vi "Filter.vi"(7 "Bandwidth":i32=2, 8 "error in (no error)":errorcluster, 9 "Frequency":i32=2, 10 "Channel index":i32=2, 11 "array":waveform(dbl)[](array[waveform])) -> (0 "error out":errorcluster, 1 "dt":dbl, 2 "Channel name":string, 3 "Amplitude":dbl)   [LabVIEW 2019]
doc: "This example demonstrates how to acquire a continuous amount of data (Waveform) using the DAQ device's internal clock. It also shows how to synchronize two devices for different device families (E Series, S Series, M Series, X Series, DSA, and SC Express), to simultaneously acquire the data.\n\nFor instructions on how to connect your signals to the DAQ device, refer to your device documentation."
uses:
  <vilib>/Waveform/WDTOps.llb/WDT Get Final Time Value DBL.vi
  <vilib>/Analysis/NI_AALPro.lvlib
panel:
  # "Filter"
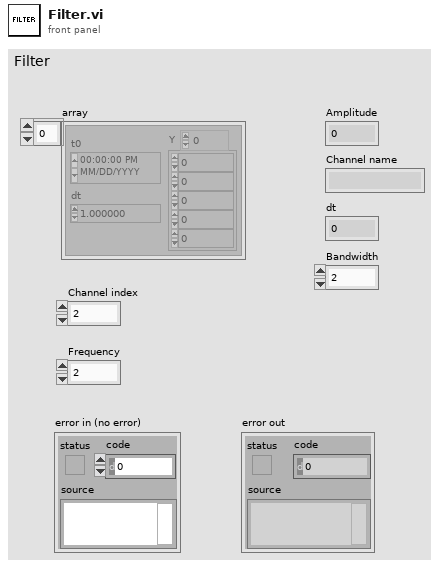
[diagram p1: front panel]
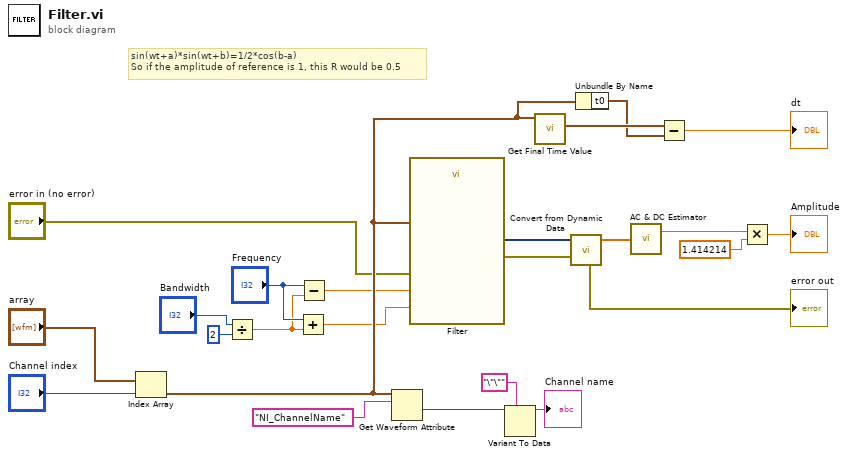
[diagram p0: block diagram]
diagram:
  # "sin(wt+a)*sin(wt+b)=1/2*cos(b-a)\nSo if the amplitude of reference is 1, this R would be 0.5"
  n1 = Index Array(array="array", index="Channel index") -> (element=w14:waveform(dbl))
  n2 = Divide(x="Bandwidth", y=2) -> (x/y=w8:dbl)
  n3 = Add(x="Frequency", y=w8) -> (x+y=w6:dbl)
  n4 = Subtract(x="Frequency", y=w8) -> (x-y=w7:dbl)
  n5 = Get Waveform Attribute(6:"NI_ChannelName" ("name"), 7:w14) -> (1:w18:variant)  [unwired: 2 in, 3 out]
  n6 = call "Filter"("error in (no error)"="error in (no error)", "Lower Cut-Off"=w7, "Upper Cut-Off"=w6, "Signal"=w14) -> ("error out"=→"error out":errorcluster, "Filtered Signal"=w5:dynamicdata)  [unwired: 6 in]
  n7 = Variant To Data(type="\"\"" ("name"), Variant=w18) -> (data=→"Channel name":string)  [unwired: 1 in, 1 out]
  n8 = call-poly <vilib>:"Get Final Time Value.vi"("waveform in"=w14) -> ("tf"=w23:timestamp)  [unwired: 8 in, 2 out]
  n9 = call "Convert from Dynamic Data"("Dynamic Data Type"=w5) -> ("Array"=w4:dbl[])  [unwired: 3 in]
  n10 = Unbundle By Name(w14) -> ("t0"=w22:timestamp)
  n11 = call <vilib>:"AC & DC Estimator.vi"("Signal (V)"=w4) -> ("AC estimate (Vrms)"=w2:dbl)  [unwired: 1 out]
  n12 = Subtract(x=w23, y=w22) -> (x-y=→"dt":dbl)
  n13 = Multiply(x=w2, y=1.414214) -> (x*y=→"Amplitude":dbl)
